vi "Report Event.vi"(7 "Event Level (Info)":T1=enum."Info", 8 "error in (no error)":errorcluster, 10 "Message":string, 11 "Vecto in":refnum<class "Vecto.lvclass">) -> (0 "error out":errorcluster, 3 "Vecto out":refnum<class "Vecto.lvclass">)   [LabVIEW 2020, in "Vecto.lvlib" / "Vecto.lvclass"]
uses:
  Vecto.lvclass
  Vecto.lvclass/Vecto.ctl
  EventLoggingService/EventLoggingService.lvclass
  Event Level.ctl
  Vecto.lvlib
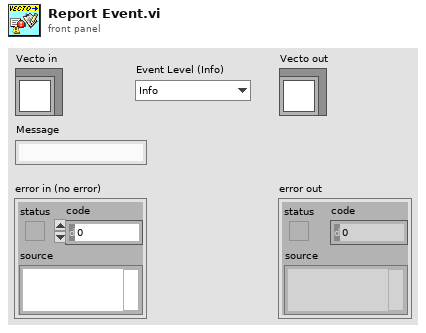
[diagram p1: front panel]
types:
  T1 = typedef "Vecto.lvlib/Event Level.ctl" = enum16{"Debug", "Info", "Warning", "Error"}
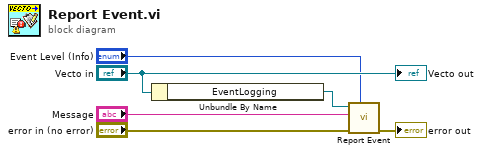
[diagram p0: block diagram]
diagram:
  n1 = Unbundle By Name("Vecto in") -> ("EventLogging"=w5:refnum<class "EventLoggingService.lvclass">)
  n2 = call "Report Event.vi"("Event Level (Info)"="Event Level (Info)", "error in (no error)"="error in (no error)", "Message"="Message", "EventLoggingService in"=w5) -> ("error out"=→"error out":errorcluster)  [unwired: 6 in, 1 out]
  "Vecto out" <- "Vecto in"
